vi "DataLogging.vi"   [LabVIEW 2017]
uses:
  <vilib>/Platform/TimedLoop/XDataNode/timing_clust.ctl
  <vilib>/Platform/TimedLoop/XDataNode/nitl_modes.ctl
  <vilib>/Platform/TimedLoop/XDataNode/wakeup.ctl
  <vilib>/platform/TimedLoop/XDataNode/XDataNode.xnode
  <vilib>/Platform/TimedLoop/XDataNode/XDNodeRunTimeDep.lvlib
types:
  T1 = enum16{"open", "open or create", "create or replace", "create", "open (read-only)"}
  T2 = typedef "XDNodeRunTimeDep.lvlib/timing_clust.ctl" = cluster{"Expected End [f-1]":u64, "Actual End [f-1]":u64, "Finished Late? [f-1]":bool, "Expected End [i-1]":u64, "Actual End [i-1]":u64, "Finished Late? [i-1]":bool, "Expected Start [i]":u64, "Actual Start [i]":u64, "Expected Start [f]":u64, "Actual Start [f]":u64, "Source Name":string, "Structure Name":string, "Period":i64, "Deadline":i64, "Offset":i64, "Start":i64, "Priority":i32, "Timeout":i32, "Mode":T3, "Wakeup Reason":T4, "Error":errorcluster, "Source Type":string, "Secondary Source Type":string, "Global End Time":u64, "Global Start Time":u64, "Frame Duration":u64, "Iteration Duration":u64, "Assigned CPU":i32, "I/O Scan Engine Mode":u32}
  T3 = typedef "XDNodeRunTimeDep.lvlib/nitl_modes.ctl" = enum32{"No Change", "Process missed periods, maintain original phase", "Discard missed periods, maintain original phase", "Process missed periods, ignore original phase", "Discard missed periods, ignore original phase"}
  T4 = typedef "XDNodeRunTimeDep.lvlib/wakeup.ctl" = enum32{"Normal", "Aborted", "Asynchronous wakeup", "Timing source error", "Timed loop error", "Timeout"}
  T5 = cluster{"Primary Battery 1 Voltage":sgl, "Primary Battery 2 Voltage":sgl, "Reserve Battery Voltage":sgl, "Primary Battery 1 Current":sgl, "Primary Battery 2 Current":sgl, "Reserve Battery Current":sgl, "Primary Battery 1 Temperature":sgl, "Primary Battery 2 Temperature":sgl, "Reserve Battery Temperature":sgl, "Primary Battery 1 Low":bool, "Primary Battery 2 Low":bool, "Reserve Battery Low":bool, "Primary Battery 1 Critical":bool, "Primary Battery 2 Critical":bool, "Reserve Battery Critical":bool, "Primary Battery 1 Hot":bool, "Primary Battery 2 Hot":bool, "Reserve Battery Hot":bool, "Frame Temperature":sgl, "Frame Hot":bool, "Ambient Pressure":sgl, "Tank Pressure":sgl, "Downstream Pressure":sgl, "Tank Pressue Low":bool, "Downstream Pressure Low":bool, "Tank Pressure Fault":bool, "Downstream Pressure Fault":bool, "IR 1 RAW":sgl, "IR 2 RAW":sgl, "IR Fault":bool, "Pusher Connected":bool, "Left Tape Count":u32, "Right Tape Count":u32, "Left Velocity":sgl, "Right Velocity":sgl, "Left LS Fault":bool, "Right LS Fault":bool, "Levitation Height":sgl, "Levitating?":bool, "PCS 1 Position":sgl, "PCS 2 Position":sgl, "PCS 3 Position":sgl, "PCS 4 Position":sgl, "FL Count":u8, "FR Count":u8, " BL Count":u8, "BR Count":u8}
  T6 = cluster{"X dtheta":sgl, "Y dtheta":sgl, "Z dtheta":sgl, "X accel":sgl, "Y accel":sgl, "Z accel":sgl, "Velocity":sgl, "IMU Fault":bool, "Time Since Last Tape":sgl, "Position":sgl}
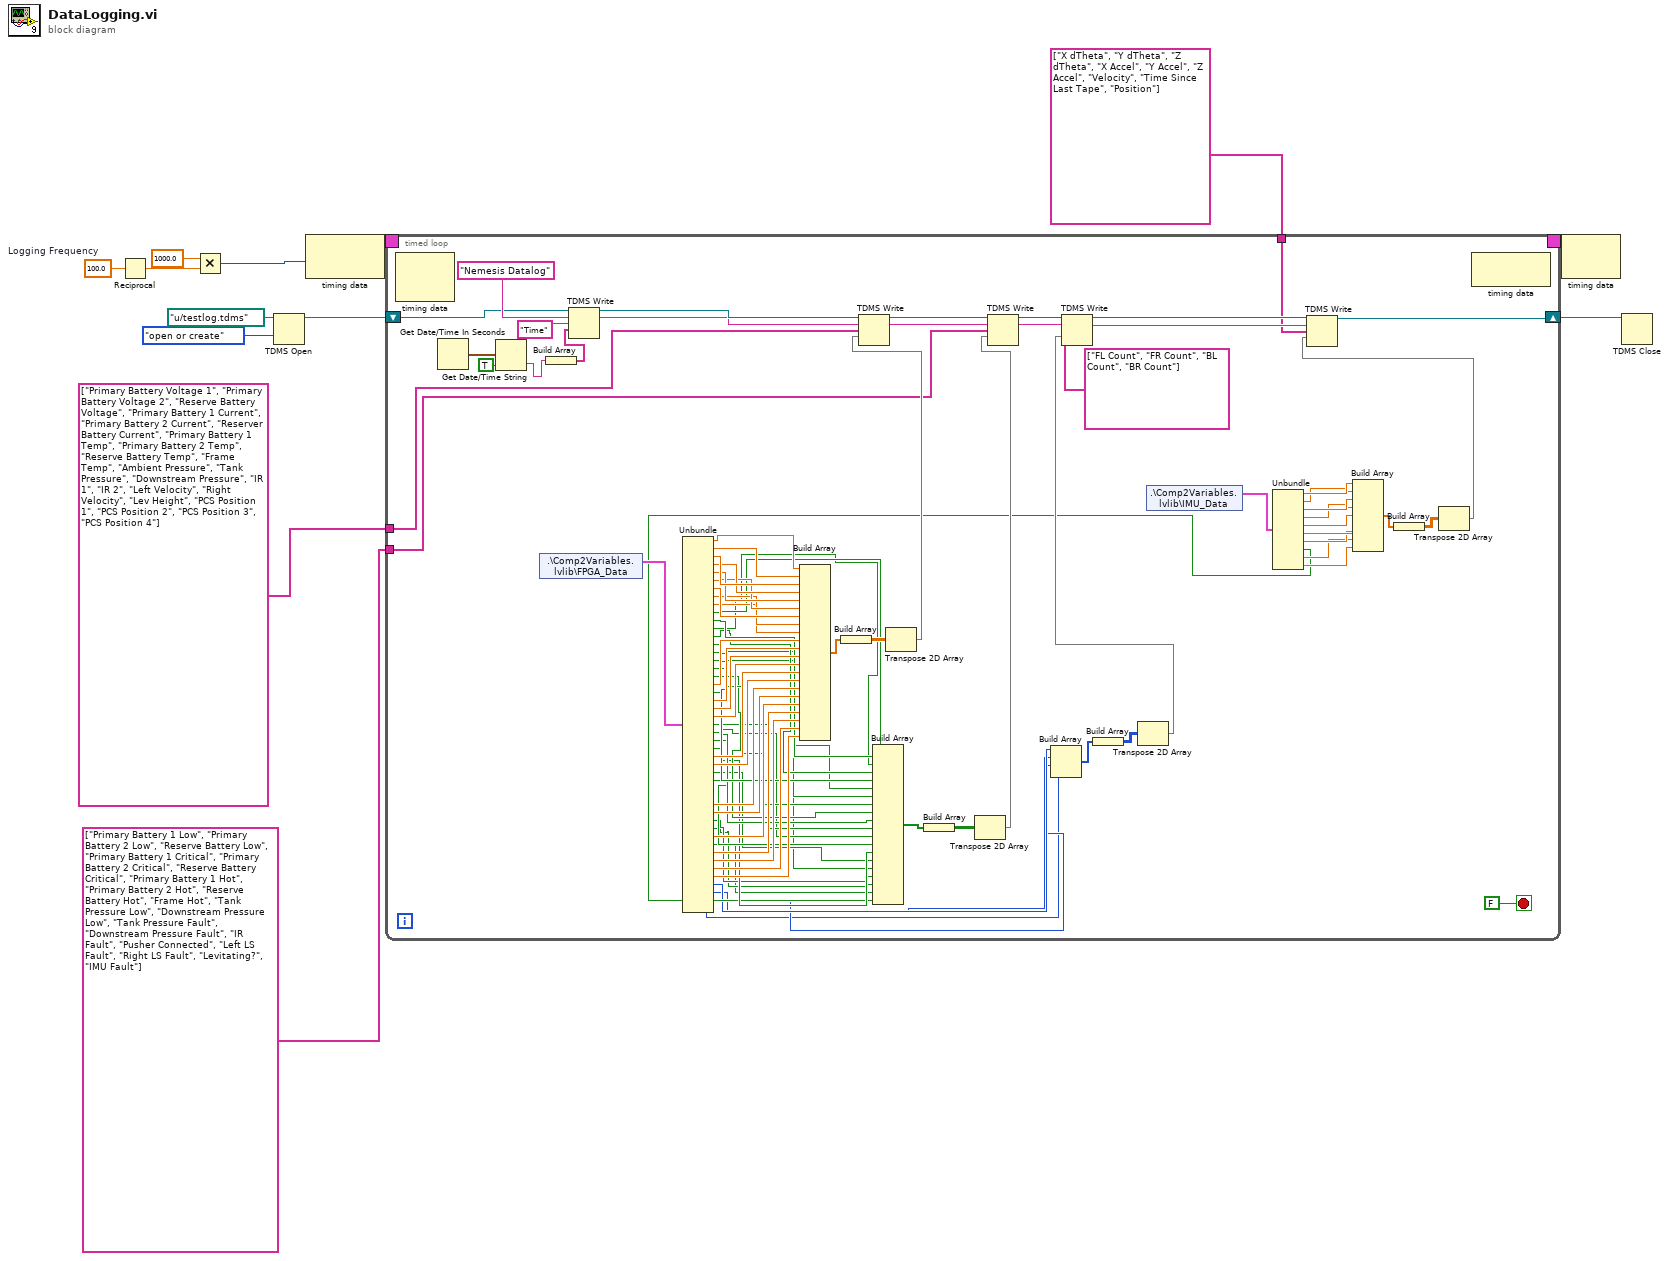
[diagram p0: block diagram]
diagram:
  w7 = 100.0  # Logging Frequency
  n1 = Reciprocal(x=w7) -> (1/x=w4:dbl)
  n2 = Multiply(x=1000.0, y=w4) -> (x*y=w6:i64)
  n3 = TDMS Open(10:T1."open or create" ("operation (0:open)"), 11:path "u:/testlog.tdms" ("file path")) -> (3:w9:refnum<k34>)  [unwired: 5 in, 1 out]
  n4 = node-c288(w6) -> (w13:T2)
  n5 = timed-loop {
    timing: w13 -> [_]
    timing-out: [_] -> w12
    shift-right: [w19] -> w11
    shift-left: w9 -> [w41]
    tunnel: string[] ["Primary Battery Voltage 1", "Primary Battery Voltage 2", "Reserve Battery Voltage", "Primary Battery 1 Current", "Primary Battery 2 Current", "Reserver Battery Current", "Primary Battery 1 Temp", "Primary Battery 2 Temp", "Reserve Battery Temp", "Frame Temp", "Ambient Pressure", "Tank Pressure", "Downstream Pressure", "IR 1", "IR 2", "Left Velocity", "Right Velocity", "Lev Height", "PCS Position 1", "PCS Position 2", "PCS Position 3", "PCS Position 4"] ("channel name(s) in (Untitled)") -> [w39]
    tunnel: string[] ["Primary Battery 1 Low", "Primary Battery 2 Low", "Reserve Battery Low", "Primary Battery 1 Critical", "Primary Battery 2 Critical", "Reserve Battery Critical", "Primary Battery 1 Hot", "Primary Battery 2 Hot", "Reserve Battery Hot", "Frame Hot", "Tank Pressure Low", "Downstream Pressure Low", "Tank Pressure Fault", "Downstream Pressure Fault", "IR Fault", "Pusher Connected", "Left LS Fault", "Right LS Fault", "Levitating?", "IMU Fault"] ("channel name(s) in (Untitled)") -> [w38]
    tunnel: string[] ["X dTheta", "Y dTheta", "Z dTheta", "X Accel", "Y Accel", "Z Accel", "Velocity", "Time Since Last Tape", "Position"] ("channel name(s) in (Untitled)") -> [w21]
    stop <- FALSE stop-if-true
    n6 = node-c288() -> ()  [unwired: 1 in, 2 out]
    n7 = Get Date/Time In Seconds() -> (seconds since 1Jan1904=w102:timestamp)
    n8 = Get Date/Time String(seconds (now)=w102, want seconds? (F)=TRUE) -> (time string=w100:string)  [unwired: 1 in, 1 out]
    n9 = shared-variable ".\\Comp2Variables.lvlib\\FPGA_Data"() -> (w40:T5)  [unwired: 1 in, 1 out]
    n10 = Build Array(w100) -> (w103:string[])
    n11 = TDMS Write(0:w41, 5:"Nemesis Datalog" ("group name in (Untitled)"), 7:"Time", 9:w103) -> (4:w74:refnum<k34>, 6:w73:string)  [unwired: 2 in, 2 out]
    n12 = Unbundle(w40) -> ("Primary Battery 1 Voltage"=w98:sgl, "Primary Battery 2 Voltage"=w97:sgl, "Reserve Battery Voltage"=w96:sgl, "Primary Battery 1 Current"=w95:sgl, "Primary Battery 2 Current"=w94:sgl, "Reserve Battery Current"=w93:sgl, "Primary Battery 1 Temperature"=w92:sgl, "Primary Battery 2 Temperature"=w91:sgl, "Reserve Battery Temperature"=w90:sgl, "Primary Battery 1 Low"=w71:bool, "Primary Battery 2 Low"=w70:bool, "Reserve Battery Low"=w69:bool, "Primary Battery 1 Critical"=w68:bool, "Primary Battery 2 Critical"=w67:bool, "Reserve Battery Critical"=w66:bool, "Primary Battery 1 Hot"=w65:bool, "Primary Battery 2 Hot"=w64:bool, "Reserve Battery Hot"=w63:bool, "Frame Temperature"=w89:sgl, "Frame Hot"=w62:bool, "Ambient Pressure"=w88:sgl, "Tank Pressure"=w87:sgl, "Downstream Pressure"=w86:sgl, "Tank Pressue Low"=w61:bool, "Downstream Pressure Low"=w60:bool, "Tank Pressure Fault"=w59:bool, "Downstream Pressure Fault"=w58:bool, "IR 1 RAW"=w85:sgl, "IR 2 RAW"=w84:sgl, "IR Fault"=w57:bool, "Pusher Connected"=w56:bool, "Left Velocity"=w83:sgl, "Right Velocity"=w82:sgl, "Left LS Fault"=w55:bool, "Right LS Fault"=w54:bool, "Levitation Height"=w81:sgl, "Levitating?"=w53:bool, "PCS 1 Position"=w80:sgl, "PCS 2 Position"=w79:sgl, "PCS 3 Position"=w78:sgl, "PCS 4 Position"=w77:sgl, "FL Count"=w18:u8, "FR Count"=w17:u8, "BL Count"=w16:u8, "BR Count"=w15:u8)  [unwired: 2 out]
    n13 = Build Array(w98, w97, w96, w95, w94, w93, w92, w91, w90, w89, w88, w87, w86, w85, w84, w83, w82, w81, w80, w79, w78, w77) -> (w75:sgl[])
    n14 = Build Array(w75) -> (w76:sgl[][])
    n15 = Transpose 2D Array(2D array=w76) -> (transposed array=w72:sgl[][])
    n16 = TDMS Write(0:w74, 5:w73, 7:w39, 9:w72) -> (4:w50:refnum<k34>, 6:w48:string)  [unwired: 2 in, 2 out]
    n17 = Build Array(w18, w17, w16, w15) -> (w47:u8[])
    n18 = Build Array(w47) -> (w46:u8[][])
    n19 = Transpose 2D Array(2D array=w46) -> (transposed array=w45:u8[][])
    n20 = shared-variable ".\\Comp2Variables.lvlib\\IMU_Data"() -> (w35:T6)  [unwired: 1 in, 1 out]
    n21 = Unbundle(w35) -> ("X dtheta"=w34:sgl, "Y dtheta"=w33:sgl, "Z dtheta"=w32:sgl, "X accel"=w31:sgl, "Y accel"=w30:sgl, "Z accel"=w29:sgl, "Velocity"=w28:sgl, "IMU Fault"=w20:bool, "Time Since Last Tape"=w27:sgl, "Position"=w26:sgl)
    n22 = Build Array(w71, w70, w69, w68, w67, w66, w65, w64, w63, w62, w61, w60, w59, w58, w57, w56, w55, w54, w53, w20) -> (w51:bool[])
    n23 = Build Array(w51) -> (w52:bool[][])
    n24 = Transpose 2D Array(2D array=w52) -> (transposed array=w49:bool[][])
    n25 = TDMS Write(0:w50, 5:w48, 7:w38, 9:w49) -> (4:w43:refnum<k34>, 6:w44:string)  [unwired: 2 in, 2 out]
    n26 = TDMS Write(0:w43, 5:w44, 7:string[] ["FL Count", "FR Count", "BL Count", "BR Count"] ("channel name(s) in (Untitled)"), 9:w45) -> (4:w36:refnum<k34>, 6:w22:string)  [unwired: 2 in, 2 out]
    n27 = Build Array(w34, w33, w32, w31, w30, w29, w28, w27, w26) -> (w24:sgl[])
    n28 = Build Array(w24) -> (w25:sgl[][])
    n29 = Transpose 2D Array(2D array=w25) -> (transposed array=w23:sgl[][])
    n30 = TDMS Write(0:w36, 5:w22, 7:w21, 9:w23) -> (4:w19:refnum<k34>)  [unwired: 2 in, 3 out]
    n31 = node-c288() -> ()  [unwired: 1 in, 1 out]
  }
  n32 = node-c288(w12) -> ()  [unwired: 1 out]
  n33 = TDMS Close(11:w11) -> ()  [unwired: 1 in, 2 out]
